vi "VI Name for window Title.vi"(8 "error in":errorcluster, 11 "vi reference":refnum<vi>) -> (0 "error out":errorcluster, 2 "Vi tiltle":string, 3 "vi reference out (dup)":refnum<vi>)   [LabVIEW 2014]
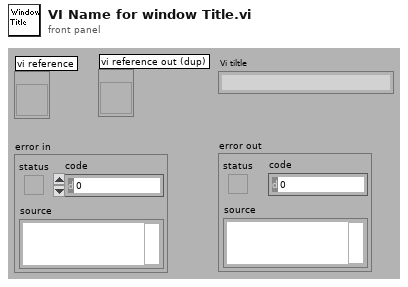
[diagram p1: front panel]
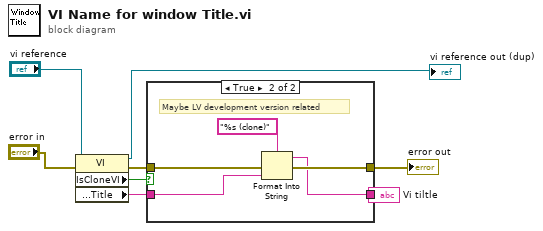
[diagram p0: block diagram]
diagram:
  n1 = property class="VI"(reference="vi reference", error in="error in") -> (reference out=→"vi reference out (dup)":refnum<vi>, error out=w4:errorcluster, "IsCloneVI"=w2:bool, "Front Panel.Title"=w6:string)
  n2 = case shown="True" w2 {
    tunnel: [w10 w13] -> w5
    tunnel: w6 -> [w10 w12]
    tunnel: w4 -> [w9 w11]
    tunnel: [w9 w14] -> w3
    frame False {
    }
    frame True {
      # "Maybe LV development version related"
      n3 = Format Into String(format string="%s (clone)", error in=w11, w12) -> (resulting string=w13:string, error out=w14:errorcluster)  [unwired: 1 in]
    }
  }
  "error out" <- w3
  "Vi tiltle" <- w5
